vi "Log.vi"(8 "error in (no error)":errorcluster, 10 "String to add":string, 11 "Actor_Log in":refnum<class "Actor_Log.lvclass">) -> (0 "error out":errorcluster, 3 "Actor_Log out":refnum<class "Actor_Log.lvclass">)   [LabVIEW 2020, in "Library Core.lvlib" / "Actor_Log.lvlib" / "Actor_Log.lvclass"]
uses:
  Actor_Log.lvclass
  Actor_Log.lvclass/Actor_Log.ctl
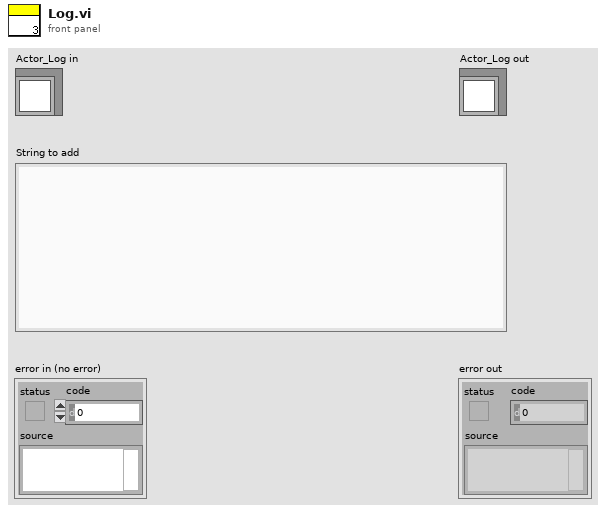
[diagram p1: front panel]
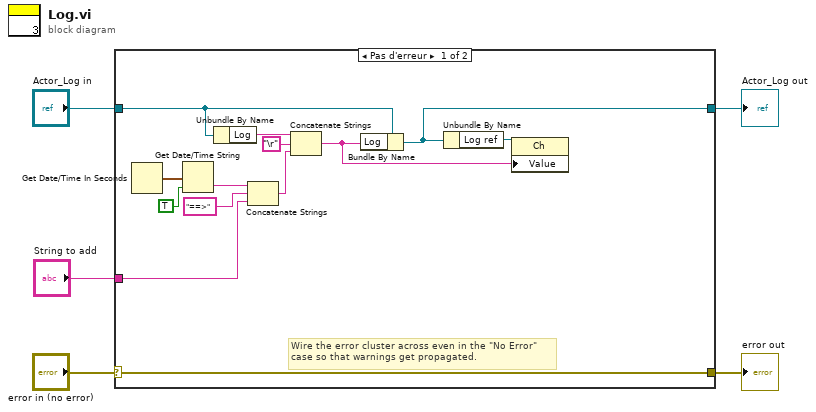
[diagram p0: block diagram]
diagram:
  n1 = case shown="Pas d'erreur" "error in (no error)" {
    selector: "error in (no error)" -> [w18 w20]
    tunnel: [w18 w20] -> w4
    tunnel: [w8 w19] -> w2
    tunnel: "Actor_Log in" -> [w9 w19]
    tunnel: "String to add" -> [w11 _]
    frame No Error {
      # "Wire the error cluster across even in the \"No Error\"\ncase so that warnings get propagated."
      n2 = Get Date/Time In Seconds() -> (seconds since 1Jan1904=w15:timestamp)
      n3 = Get Date/Time String(seconds (now)=w15, want seconds? (F)=TRUE) -> (time string=w13:string)  [unwired: 1 in, 1 out]
      n4 = Unbundle By Name(w9) -> ("Log"=w17:string)
      n5 = Concatenate Strings(w13, "==>", w11) -> (w10:string)
      n6 = Concatenate Strings(w17, "\r", w10) -> (w6:string)
      n7 = Bundle By Name(cluster=w9, "Log"=w6) -> (w8:refnum<class "Actor_Log.lvclass">)
      n8 = Unbundle By Name(w8) -> ("Log ref"=w7:refnum<vi>)
      n9 = property class="Ch"(reference=w7, "Value"=w6) -> ()  [unwired: 1 in, 2 out]
    }
    frame Error {
    }
  }
  "error out" <- w4
  "Actor_Log out" <- w2
